vi "Wrap g-CLI.vi"(8 "error in (no error)":errorcluster {"code" format="Error %.0f"}, 11 "CLI":refnum<class "CLI.lvclass">) -> (0 "error out":errorcluster {"code" format="Error %.0f"}, 3 "g-CLI Interaction out":refnum<class "g-CLI Interaction.lvclass">)   [LabVIEW 2023, in "g-CLI Interaction.lvclass"]
uses:
  g-CLI Interaction.lvclass
  <vilib>/Wiresmith Technology/G CLI/CLI Class/CLI.lvclass
  g-CLI Interaction.lvclass/g-CLI Interaction.ctl
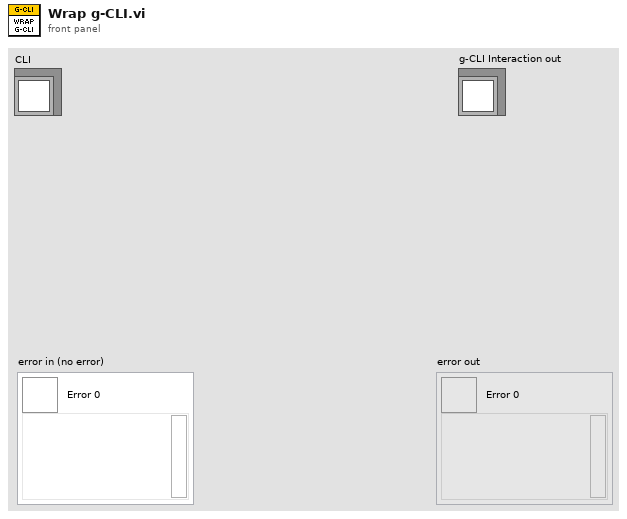
[diagram p1: front panel]
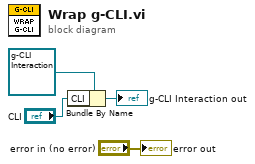
[diagram p0: block diagram]
diagram:
  n1 = Bundle By Name(cluster=refnum<class "g-CLI Interaction.lvclass"> refnum ("g-CLI Interaction out"), "CLI"="CLI") -> (→"g-CLI Interaction out":refnum<class "g-CLI Interaction.lvclass">)
  "error out" <- "error in (no error)"
